vi "Sub VI.vi"() -> ()   [LabVIEW 2016]
panel:
  out "main Graph 2":waveform(dbl)[](graph)
  out "Numeric":i32
  in  "stop":bool
  # "This is a mock new window"
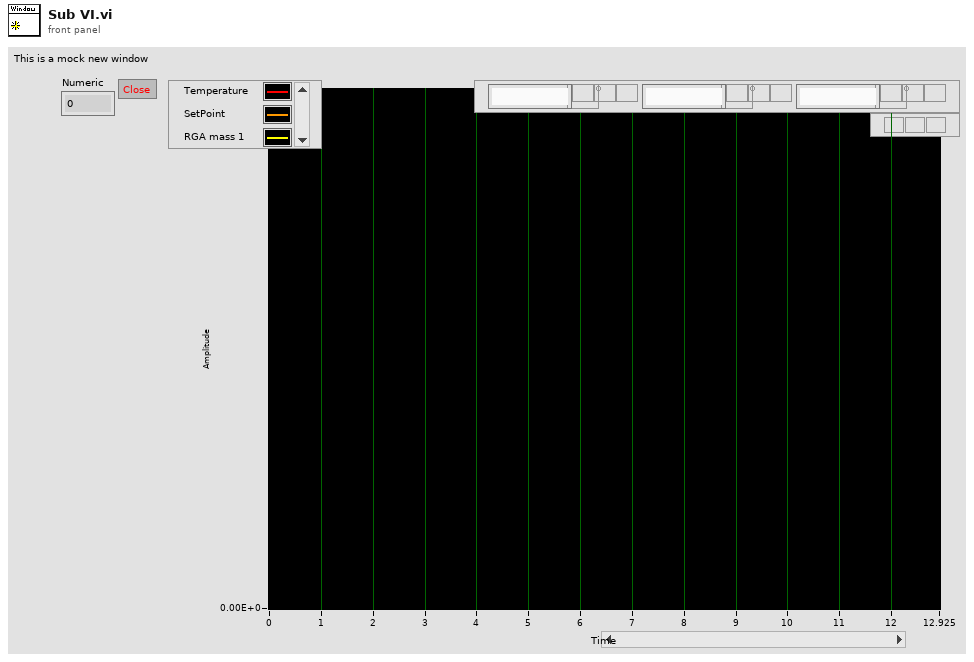
[diagram p1: front panel]
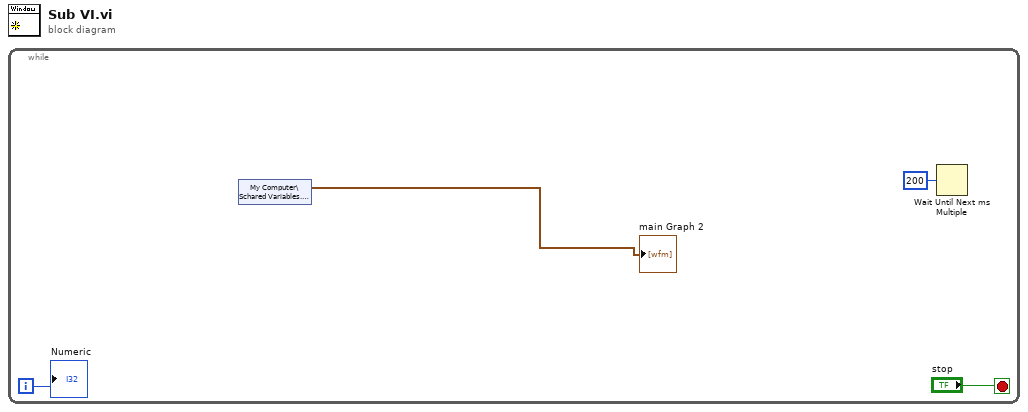
[diagram p0: block diagram]
diagram:
  n1 = while {
    i -> [w2]
    stop <- "stop" stop-if-true
    n2 = shared-variable "My Computer\\Schared Variables.lvlib\\Array"() -> (→"main Graph 2":waveform(dbl)[])  [unwired: 1 in, 1 out]
    n3 = Wait Until Next ms Multiple(millisecond multiple=u32 200) -> ()  [unwired: 1 out]
    "Numeric" <- w2
  }
